vi "Connect - Instrument with Channel(s).vi"(8 "error in (no error)":errorcluster, 10 "Channel(s)":i32[](array[numeric]), 11 "PXIe5413 in":refnum<class "PXIe5413.lvclass">) -> (0 "error out":errorcluster, 3 "PXIe5413 out":refnum<class "PXIe5413.lvclass">)   [LabVIEW 2018, in "PXIe5413.lvlib" / "PXIe5413.lvclass"]
uses:
  PXIe5413.lvclass
  PXIe5413.lvclass/PXIe5413.ctl
  PPLs/Function Generator/Parent/Function Generator.lvlibp/Function Generator.lvclass
  C:/Projects/LabVIEW/PPLs/Function Generator/Parent/Function Generator.lvlibp/Function Generator.lvclass
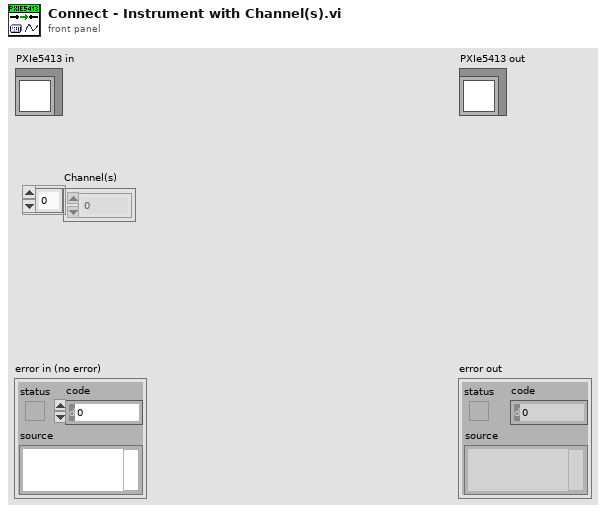
[diagram p1: front panel]
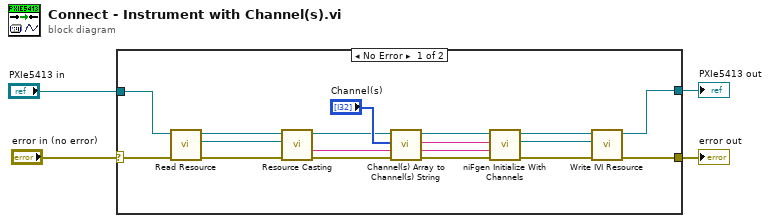
[diagram p0: block diagram]
diagram:
  n1 = case shown="No Error" "error in (no error)" {
    selector: "error in (no error)" -> [w16 w22]
    tunnel: [w5 w22] -> w3
    tunnel: [w7 w21] -> w2
    tunnel: "PXIe5413 in" -> [w17 w21]
    frame No Error {
      n2 = call "Read Resource.vi"("error in (no error)"=w16, "Function Generator in"=w17) -> ("error out"=w20:errorcluster, "Resource"=w10:refnum<visa-resource-name>, "Function Generator out"=w19:refnum<class "PXIe5413.lvclass">)  [unwired: 7 in]
      n3 = call "Resource Casting.vi"("error in (no error)"=w20, "VISA Resource In"=w10, "PXIe5413 in"=w19) -> ("error out"=w13:errorcluster, "Casted Resource"=w18:string, "PXIe5413 out"=w14:refnum<class "PXIe5413.lvclass">)  [unwired: 6 in]
      n4 = call "Channel(s) Array to Channel(s) String.vi"("error in (no error)"=w13, "Channel(s)"="Channel(s)", "PXIe5413 in"=w14) -> ("error out"=w12:errorcluster, "Channels String"=w11:string, "PXIe5413 out"=w8:refnum<class "PXIe5413.lvclass">)  [unwired: 6 in]
      n5 = call <instrlib>:"niFgen Initialize With Channels.vi"("error in (no error)"=w12, "Channel Name"=w11, "Resource Name"=w18) -> ("error out"=w6:errorcluster, "Instrument Handle Out"=w9:refnum<k15>)  [unwired: 7 in]
      n6 = call "Write IVI Resource.vi"("error in (no error)"=w6, "IVI Resource"=w9, "PXIe5413 in"=w8) -> ("error out"=w5:errorcluster, "PXIe5413 out"=w7:refnum<class "PXIe5413.lvclass">)  [unwired: 7 in]
    }
    frame Error {
    }
  }
  "error out" <- w3
  "PXIe5413 out" <- w2
